vi "ACT_Loop.vi"() -> ()   [LabVIEW 2023, in "2024 AdPivotArm_ACT.lvlib"]
uses:
  2024 AdPivotArm_ACT.lvlib
  Cluster_CMD_ACT_Data.ctl
  Shared Code/TypeDefs/ENUM_Extend_CMD_Mode Select.ctl
  Shared Code/TypeDefs/Cluster_Extend_Config HW Values.ctl
  Shared Code/TypeDefs/Cluser_CAN Data.ctl
  Shared Code/TypeDefs/Cluster_Config FX Motor Output.ctl
  <vilib>/Rock Robotics/WPI/ThirdParty/Phoenix-LabVIEW/Motor Controller/Controls/CTRE_Phoenix_MotorControl_TalonFXInvertType.ctl
  <vilib>/Rock Robotics/WPI/ThirdParty/Phoenix-LabVIEW/Motor Controller/Controls/CTRE_Phoenix_MotorControl_NeutralMode.ctl
  Shared Code/TypeDefs/Cluster_FWD  REV Values.ctl
  Shared Code/TypeDefs/Cluster_FX SLOT PID Config.ctl
  Shared Code/TypeDefs/Cluster_PID Gains.ctl
  Shared Code/TypeDefs/Cluster_FX Motion Magic Parameters.ctl
  Shared Code/TypeDefs/Cluser_FX Config_Limit Travel.ctl
  Shared Code/TypeDefs/Cluser_Hard Limits.ctl
  <vilib>/Rock Robotics/WPI/ThirdParty/Phoenix-LabVIEW/Motor Controller/Controls/CTRE_Phoenix_MotorControl_LimitSwitchNormal.ctl
  Shared Code/TypeDefs/Cluser_Config_Soft Limits.ctl
  Shared Code/TypeDefs/Cluser_Enable-Value I32.ctl
  Shared Code/TypeDefs/Cluser_FX Config_Current Limits.ctl
  Shared Code/TypeDefs/Cluster_Cancoder_Config Data.ctl
  Shared Code/TypeDefs/Cluster_Extend HW Outputs.ctl
  Shared Code/TypeDefs/Cluster_FX CloseLoop Values.ctl
  Shared Code/TypeDefs/Cluster_FX Limit Switchs.ctl
  Shared Code/TypeDefs/Cluster_FX Current Values.ctl
  Shared Code/TypeDefs/Cluster_FX Sensor Values.ctl
  Shared Code/TypeDefs/Cluster_FX Integrated Sensor Values.ctl
  Shared Code/TypeDefs/Cluster_Extend_Config SW Values.ctl
  ENUM_ACT_State.ctl
  Shared Code/TypeDefs/Cluster_Extend_SW Output Data.ctl
  <vilib>/Rock Robotics/WPI/MotorControl/WPI_MotorControlDeviceRef.ctl
  <vilib>/Rock Robotics/WPI/MotorControl/WPI_MotorControlType.ctl
  <vilib>/Rock Robotics/SystemInterfaces/DIO/FPGA_DIOPWMChannel.ctl
  <vilib>/Rock Robotics/WPI/PWM/WPI_PWMDeadband.ctl
  <vilib>/Rock Robotics/SystemInterfaces/DIO/FPGA_DIOChannel.ctl
  <vilib>/Rock Robotics/WPI/ThirdParty/Phoenix-LabVIEW/Motor Controller/Controls/CTRE_Phoenix_MotorControl_ControlMode.ctl
  <vilib>/Rock Robotics/WPI/ThirdParty/Phoenix-LabVIEW/CANCoder/Controls/CTRE_Phoenix_CANcoder_DeviceRef.ctl
  ENUM_ACT_Action.ctl
  04ee53c9-9b63-4246-8662-e0753b0c7ce8.vi
  59f07e0f-2f3e-411b-a9d4-f777b7e34f70.vi
  d67cbdc1-c35e-4f58-b6c3-7121fa6e24ba.vi
  267fcfdb-c0dc-47c1-88bc-4cfe90507065.vi
  b5508d6c-c1cc-4273-80c5-2077d34e1483.vi
  5f725c2a-0ce1-4524-8967-e83b15fdce90.vi
  89b44e99-2ed6-4dfc-a998-459b3a1fdd77.vi
  6cc16fe4-e2d9-446e-a92a-5a1cdf729577.vi
  90b56285-4e1a-4408-995a-2e9e279006c2.vi
  <vilib>/Utility/error.llb/Trim Whitespace.vi
  5f725c2a-0ce1-4524-8967-e83b15fdce90.vi/958b2683-dd4b-41b7-8ed1-41c95f63cef0.vi
  5f725c2a-0ce1-4524-8967-e83b15fdce90.vi/95f5fa9b-6175-4b34-88ee-cece92c38279.vi
  89b44e99-2ed6-4dfc-a998-459b3a1fdd77.vi/958b2683-dd4b-41b7-8ed1-41c95f63cef0.vi
  89b44e99-2ed6-4dfc-a998-459b3a1fdd77.vi/95f5fa9b-6175-4b34-88ee-cece92c38279.vi
  6cc16fe4-e2d9-446e-a92a-5a1cdf729577.vi/958b2683-dd4b-41b7-8ed1-41c95f63cef0.vi
  6cc16fe4-e2d9-446e-a92a-5a1cdf729577.vi/95f5fa9b-6175-4b34-88ee-cece92c38279.vi
  90b56285-4e1a-4408-995a-2e9e279006c2.vi/958b2683-dd4b-41b7-8ed1-41c95f63cef0.vi
  90b56285-4e1a-4408-995a-2e9e279006c2.vi/95f5fa9b-6175-4b34-88ee-cece92c38279.vi
  <vilib>/Utility/error.llb/Trim Whitespace One-Sided.vi
  5f725c2a-0ce1-4524-8967-e83b15fdce90.vi/95f5fa9b-6175-4b34-88ee-cece92c38279.vi/1c6bd52c-bbca-4d4a-a290-93ea2703fded.vi
  5f725c2a-0ce1-4524-8967-e83b15fdce90.vi/95f5fa9b-6175-4b34-88ee-cece92c38279.vi/47c2b0d5-b5fa-444e-9535-611565d375db.vi
  89b44e99-2ed6-4dfc-a998-459b3a1fdd77.vi/95f5fa9b-6175-4b34-88ee-cece92c38279.vi/1c6bd52c-bbca-4d4a-a290-93ea2703fded.vi
  89b44e99-2ed6-4dfc-a998-459b3a1fdd77.vi/95f5fa9b-6175-4b34-88ee-cece92c38279.vi/47c2b0d5-b5fa-444e-9535-611565d375db.vi
  6cc16fe4-e2d9-446e-a92a-5a1cdf729577.vi/95f5fa9b-6175-4b34-88ee-cece92c38279.vi/1c6bd52c-bbca-4d4a-a290-93ea2703fded.vi
  6cc16fe4-e2d9-446e-a92a-5a1cdf729577.vi/95f5fa9b-6175-4b34-88ee-cece92c38279.vi/47c2b0d5-b5fa-444e-9535-611565d375db.vi
  90b56285-4e1a-4408-995a-2e9e279006c2.vi/95f5fa9b-6175-4b34-88ee-cece92c38279.vi/1c6bd52c-bbca-4d4a-a290-93ea2703fded.vi
  90b56285-4e1a-4408-995a-2e9e279006c2.vi/95f5fa9b-6175-4b34-88ee-cece92c38279.vi/47c2b0d5-b5fa-444e-9535-611565d375db.vi
  RoboRIO Utilities/Global_STOP.vi
  Global_CMD_ACT_Data In.vi
  <vilib>/Utility/Data Type/Get Type Information.vi
  Shared Code/Utility/RWA/RWA/File/RWA_PC FIle Read String.vi
  Shared Code/Utility/RWA/RWA/Read Write Anything/RWA_File String.vi
  Shared Code/Utility/RWA/RWA/File/RWA_PC File Write String.vi
  <vilib>/Rock Robotics/WPI/ThirdParty/Phoenix-LabVIEW/CANCoder/Set/CTRE_Phoenix_CANcoder_SetPosition.vi
  Global_ACT_Data Out.vi
  <vilib>/Comparison/Equal/Equal Functor/Equal Functor.lvclass
panel:
  in  "CMD Override":T1(tab)
  in  "Velocity":dbl(slide) scale=-0.3..0.3
  in  "Target Counts":i32
  in  "Positon GO":bool
  out "Current Time":timestamp
  out "SW Outputs":T2
  out "Sensor Read time":dbl format="%.3f"
  in  "Force Home":bool
  out "State":T3
  in  "SW Config":T4={"ExtendSW Ver"=0, "Home Speed (0-1)"=0.2, "Enable Current Limit On Homing"=FALSE, "At Position Delay(S)"=0.2}
  out "HW Outputs":T5
  in  "Read Saved Config":bool
  in  "Update Config":bool
  in  "HW Config":T11={"ExtendHW Ver"=0, "CAN"={"ID"=11, "Bus"=""}, "Output"={"Type"=enum."Counter-Clockwise", "Neutral"=enum."Override to Coast", "Max"={"FWD"=1.0, "REV"=-1.0}, "Min"={"FWD"=0.0, "REV"=0.0}, "OL Ramp Rate (S)"=0.0, "Dead Band"=0.0, "CL Ramp Rate (S)"=0.0}, "CL"={"Gains"={"P"=1.0, "I"=0.01, "D"=0.0, "F"=0.0}, "Error Allowed"=0.0, "I Zone"=0.0, "Peak Out 0-1"=10000.0, "Max I Accu"=-1000.0}, "MM"={"Cruise Velocity"=5000, "Acceleration"=5000}, "TravelLimits"={"Hard"={"FWD Switch Normal"=enum."Normally Open", "FWD On will Zero Encoder "=FALSE, "REV Switch Normal"=enum."Normally Open", "REV On will Zero Encoder "=FALSE}, "Soft"={"FWD"={"Enable"=FALSE, "Counts"=0}, "REV"={"Enable"=FALSE, "Counts"=0}}}, "StatorLimit"={"Enable"=FALSE, "Current Limit"=0.0, "Threshold Current"=0.0, "Threshold Time"=0.0}, "Cancoder"={"ID"=0, "CW(t) CCW(f)"=TRUE, "Zero Offset"=0.0}} {"TravelLimits"."Soft"."REV"."Counts" format="%#.0f"; "TravelLimits"."Soft"."FWD"."Counts" format="%#.0f"; "Output"."Min"."REV" format="%.2f"; "Output"."Min"."FWD" format="%.2f"; "Output"."Max"."REV" format="%.2f"; "Output"."Max"."FWD" format="%.2f"; "CL"."Gains"."F" format="%#.8f"; "CL"."Gains"."D" format="%#.8f"; "CL"."Gains"."I" format="%#.8f"; "CL"."Gains"."P" format="%#.8f"}
  out "CMD":T27
  out "Cycle Time (S)":dbl format="%.3g"
  # "Teleop or Auto"
  # "STOP"
  # "Tune Output\nto 1023 Max"
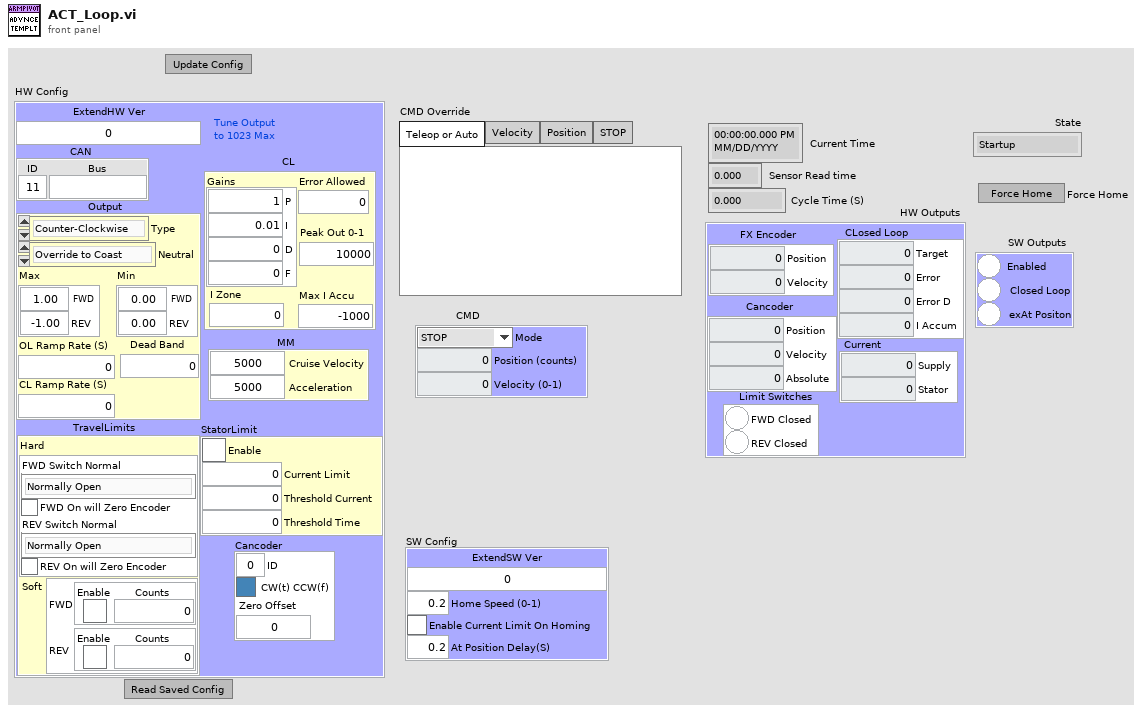
[diagram p1: front panel]
types:
  T1 = enum32{"Teleop or Auto", "Velocity", "Position", "STOP"}
  T2 = typedef "Cluster_Extend_SW Output Data.ctl" = cluster{"Enabled":bool, "Closed Loop":bool, "exAt Positon":bool}
  T3 = typedef "2024 AdPivotArm_ACT.lvlib/ENUM_ACT_State.ctl" = enum16{"Startup", "Configuring", "Stopping", "Moving Position", "Shutdown", "Homing", "Moving Velocity"}
  T4 = typedef "Cluster_Extend_Config SW Values.ctl" = cluster{"ExtendSW Ver":u64, "Home Speed (0-1)":dbl, "Enable Current Limit On Homing":bool, "At Position Delay(S)":dbl}
  T5 = typedef "Cluster_Extend HW Outputs.ctl" = cluster{"CLosed Loop":T6, "Limit Switches":T7, "Current":T8, "FX Encoder":T9, "Cancoder":T10}
  T6 = typedef "Cluster_FX CloseLoop Values.ctl" = cluster{"Target":dbl, "Error":i32, "Error D":dbl, "I Accum":dbl}
  T7 = typedef "Cluster_FX Limit Switchs.ctl" = cluster{"FWD Closed":bool, "REV Closed":bool}
  T8 = typedef "Cluster_FX Current Values.ctl" = cluster{"Supply":dbl, "Stator":dbl}
  T9 = typedef "Cluster_FX Sensor Values.ctl" = cluster{"Position":i32, "Velocity":i32}
  T10 = typedef "Cluster_FX Integrated Sensor Values.ctl" = cluster{"Position":dbl, "Velocity":dbl, "Absolute":dbl}
  T11 = typedef "Cluster_Extend_Config HW Values.ctl" = cluster{"ExtendHW Ver":u64, "CAN":T12, "Output":T13, "CL":T17, "MM":T19, "TravelLimits":T20, "StatorLimit":T25, "Cancoder":T26}
  T12 = typedef "Cluser_CAN Data.ctl" = cluster{"ID":u8, "Bus":string}
  T13 = typedef "Cluster_Config FX Motor Output.ctl" = cluster{"Type":T14, "Neutral":T15, "Max":T16, "Min":T16, "OL Ramp Rate (S)":dbl, "Dead Band":dbl, "CL Ramp Rate (S)":dbl}
  T14 = typedef "CTRE_Phoenix_MotorControl_TalonFXInvertType.ctl" = enum16{"Counter-Clockwise", "Clockwise"}
  T15 = typedef "CTRE_Phoenix_MotorControl_NeutralMode.ctl" = enum8{"EEPROMSetting", "Override to Coast", "Override to Brake"}
  T16 = typedef "Cluster_FWD  REV Values.ctl" = cluster{"FWD":dbl, "REV":dbl}
  T17 = typedef "Cluster_FX SLOT PID Config.ctl" = cluster{"Gains":T18, "Error Allowed":dbl, "I Zone":dbl, "Peak Out 0-1":dbl, "Max I Accu":dbl}
  T18 = typedef "Cluster_PID Gains.ctl" = cluster{"P":dbl, "I":dbl, "D":dbl, "F":dbl}
  T19 = typedef "Cluster_FX Motion Magic Parameters.ctl" = cluster{"Cruise Velocity":i32, "Acceleration":i32}
  T20 = typedef "Cluser_FX Config_Limit Travel.ctl" = cluster{"Hard":T21, "Soft":T23}
  T21 = typedef "Cluser_Hard Limits.ctl" = cluster{"FWD Switch Normal":T22, "FWD On will Zero Encoder ":bool, "REV Switch Normal":T22, "REV On will Zero Encoder ":bool}
  T22 = typedef "CTRE_Phoenix_MotorControl_LimitSwitchNormal.ctl" = enum16{"Normally Open", "Normally Closed", "Disabled"}
  T23 = typedef "Cluser_Config_Soft Limits.ctl" = cluster{"FWD":T24, "REV":T24}
  T24 = typedef "Cluser_Enable-Value I32.ctl" = cluster{"Enable":bool, "Counts":i32}
  T25 = typedef "Cluser_FX Config_Current Limits.ctl" = cluster{"Enable":bool, "Current Limit":dbl, "Threshold Current":dbl, "Threshold Time":dbl}
  T26 = typedef "Cluster_Cancoder_Config Data.ctl" = cluster{"ID":u8, "CW(t) CCW(f)":bool, "Zero Offset":dbl}
  T27 = typedef "2024 AdPivotArm_ACT.lvlib/Cluster_CMD_ACT_Data.ctl" = cluster{"Mode":T28, "Position (counts)":i32, "Velocity (0-1)":dbl}
  T28 = typedef "ENUM_Extend_CMD_Mode Select.ctl" = enum16{"STOP", "Position", "Velocity", "Force Home"}
  T29 = typedef "CTRE_Phoenix_CANcoder_DeviceRef.ctl" = cluster{"DeviceStatus":errorcluster, "Device Number":u8, "Handle":u64, "UsageFrame":u32, "Library Path":path}
  T30 = typedef "CTRE_Phoenix_MotorControl_ControlMode.ctl" = u16
  T31 = typedef "WPI_MotorControlDeviceRef.ctl" = cluster{"DeviceStatus":errorcluster, "Type":T32, "PWM":cluster{"PWM Channel":T33, "DeadBand":T34}, "CAN":cluster{"Device Number":u8, "SetOutput VI Ref":variant, "GetOutput VI Ref":variant, "Enable VI Ref":variant, "Disable VI Ref":variant, "Data":variant}, "Invert":bool, "DIO PWM":cluster{"PWM \"Enable\" Channel":T33, "DIOChannel":T35, "PWM Rate":dbl}}
  T32 = typedef "WPI_MotorControlType.ctl" = enum16{"PWM", "CAN", "DIO PWM"}
  T33 = typedef "FPGA_DIOPWMChannel.ctl" = enum8{"PWM 0", "PWM 1", "PWM 2", "PWM 3", "PWM 4", "PWM 5", "PWM 6", "PWM 7", "PWM 8", "PWM 9", "PWM MXP 0", "PWM MXP 1", "PWM MXP 2", "PWM MXP 3", "PWM MXP 4", "PWM MXP 5", "PWM MXP 6", "PWM MXP 7", "PWM MXP 8", "PWM MXP 9", "Invalid"}
  T34 = typedef "WPI_PWMDeadband.ctl" = cluster{"Name":string, "maxPositivePwm":i32, "minPositivePwm":i32, "centerPwm":i32, "maxNegativePwm":i32, "minNegativePwm":i32, "angularRange":u16}
  T35 = typedef "FPGA_DIOChannel.ctl" = enum8{"DIO 0", "DIO 1", "DIO 2", "DIO 3", "DIO 4", "DIO 5", "DIO 6", "DIO 7", "DIO 8", "DIO 9", "DIO MXP 0", "DIO MXP 1", "DIO MXP 2", "DIO MXP 3", "DIO MXP 4", "DIO MXP 5", "DIO MXP 6", "DIO MXP 7", "DIO MXP 8", "DIO MXP 9", "DIO MXP 10", "DIO MXP 11", "DIO MXP 12", "DIO MXP 13", "DIO MXP 14", "DIO MXP 15", "SPI Port CS1", "SPI Port CS2", "SPI Port CS3", "SPI Port MISO", "SPI Port MOSI", "Invalid"}
  T36 = cluster{"Falcon Ref":T31, "State":T3, "Previous State":T3, "Current Time":timestamp, "Previous Time":timestamp, "Start Time":timestamp, "Target Time (ms)":u32, "Cycle Time(S)":dbl, "ACT Input":T27, "ACT Output DBL":dbl, "Team Files Folder":path, "HW Config":T11, "Update Display":bool, "Max # Of Config Tries":i32, "CAN Timeout":u32, "FX Mode":T30, "FX Set Value":dbl, "HW Outputs":T5, "SW Config":T4, "SW Outputs":T2, "CANcoder Ref":T29, "Found Home":bool}
  T37 = typedef "2024 AdPivotArm_ACT.lvlib/ENUM_ACT_Action.ctl" = enum16{"No Action", "Reset Time", "Reset All", "Config HW File Read", "Config HW File Save", "Config SW File Read", "Config SW File Save", "Config From FP", "Config HW Extract", "Config HW Set", "Open HW Only", "Control FX Stop", "Control FX Home", "Control FX Motion Magic", "Control FX Speed", "Config Disable FX Soft Limit", "Config Enable FX Soft Limit", "Config HW Enable Current Limit", "Config HW Disable Current Limit", "Encoder Set to Zero", "Control FX Position", "Move to Reverse Limit "}
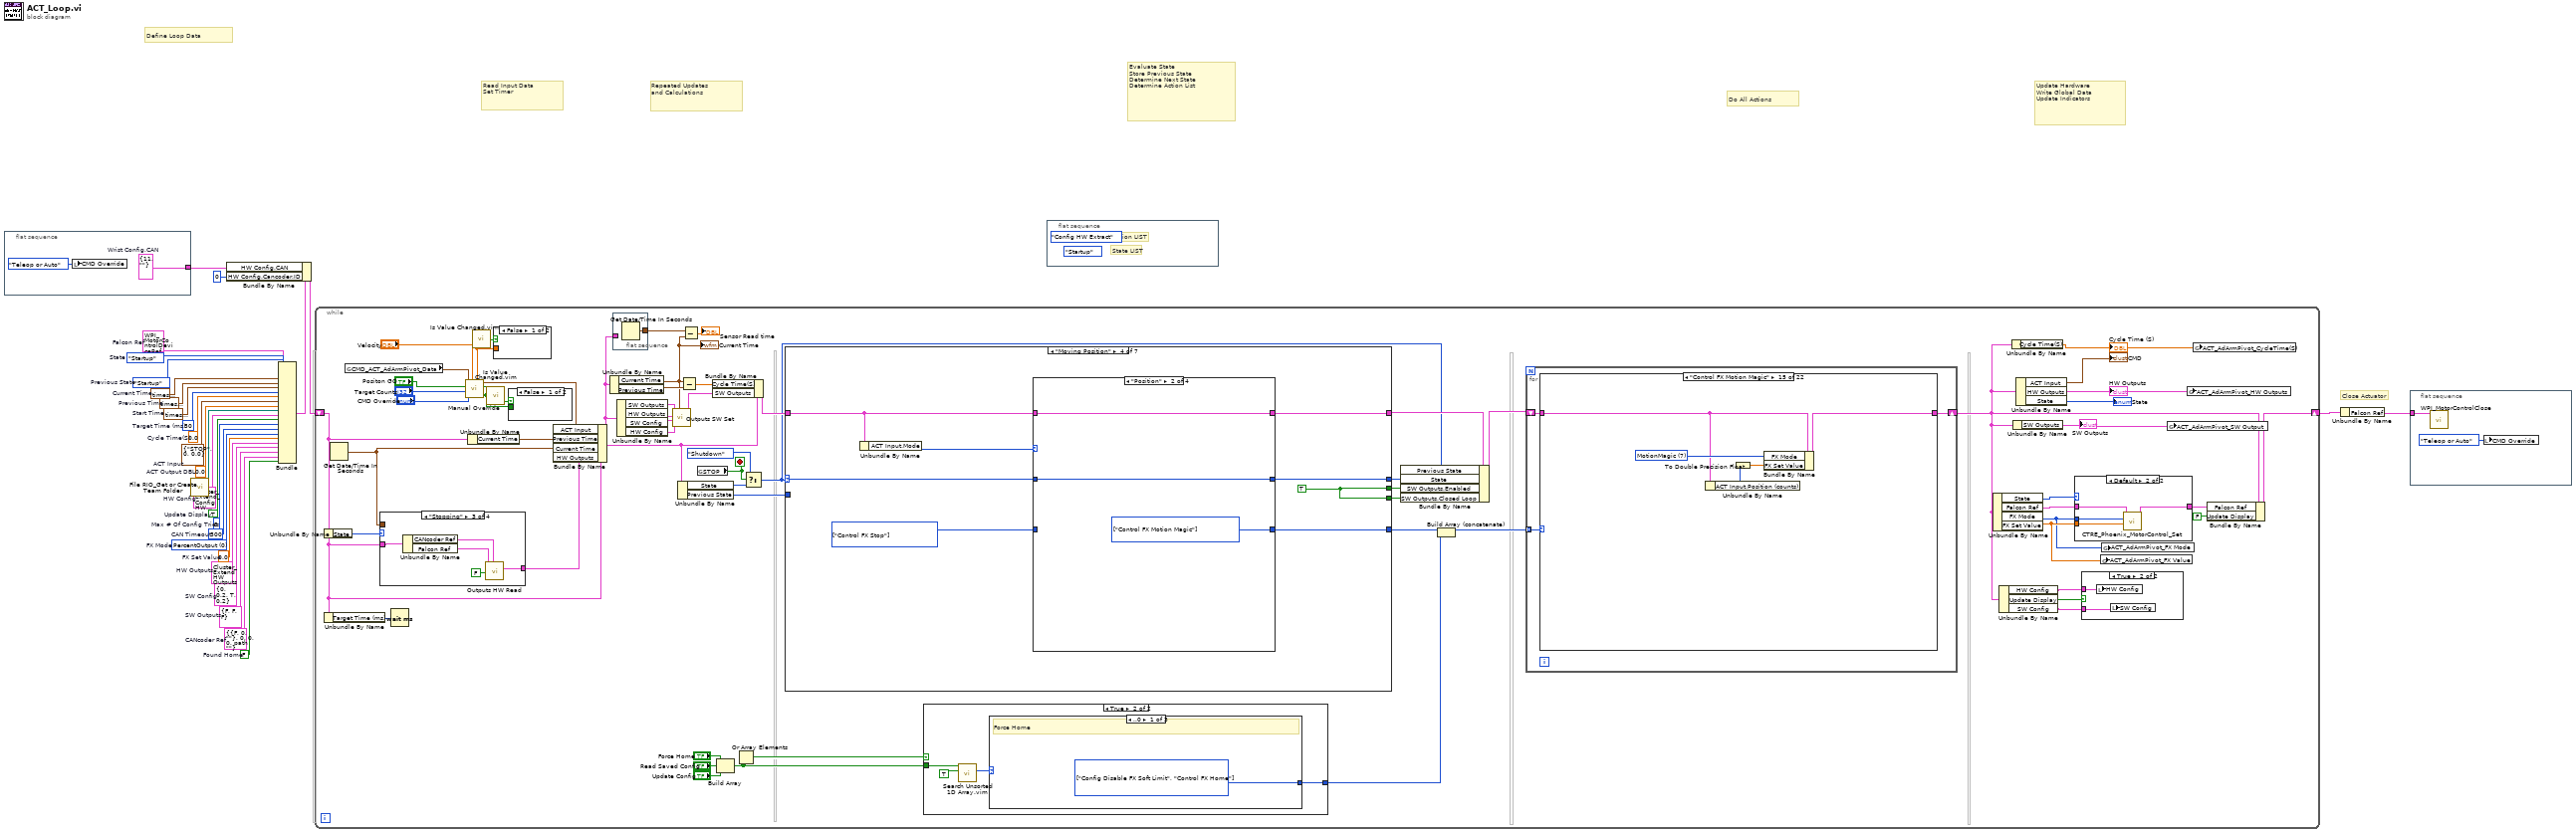
[diagram p0: block diagram]
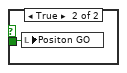
[diagram p2: hidden frame]
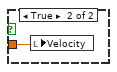
[diagram p3: hidden frame]
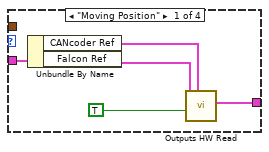
[diagram p4: hidden frame]
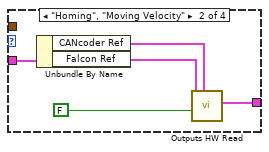
[diagram p5: hidden frame]
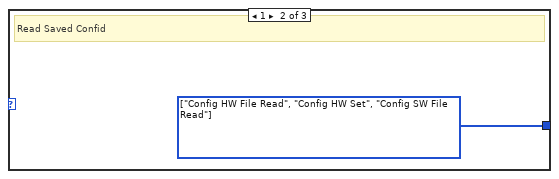
[diagram p8: hidden frame]
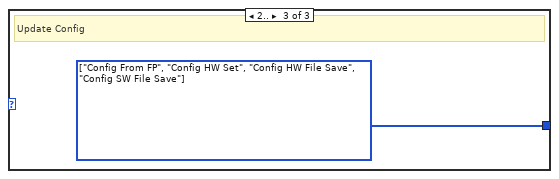
[diagram p9: hidden frame]
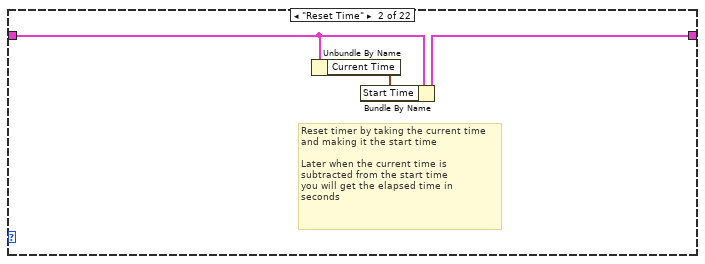
[diagram p13: hidden frame]
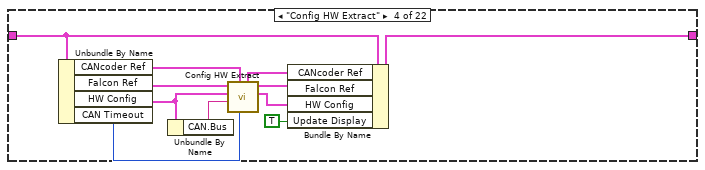
[diagram p15: hidden frame]
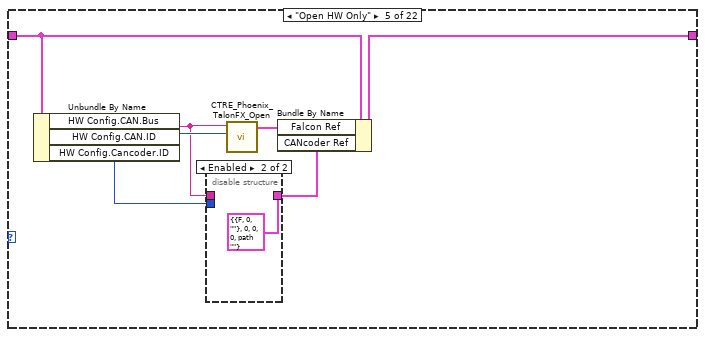
[diagram p16: hidden frame]
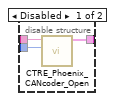
[diagram p17: hidden frame]
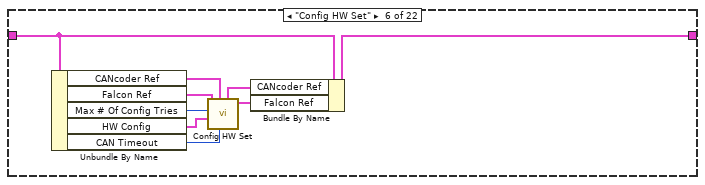
[diagram p18: hidden frame]
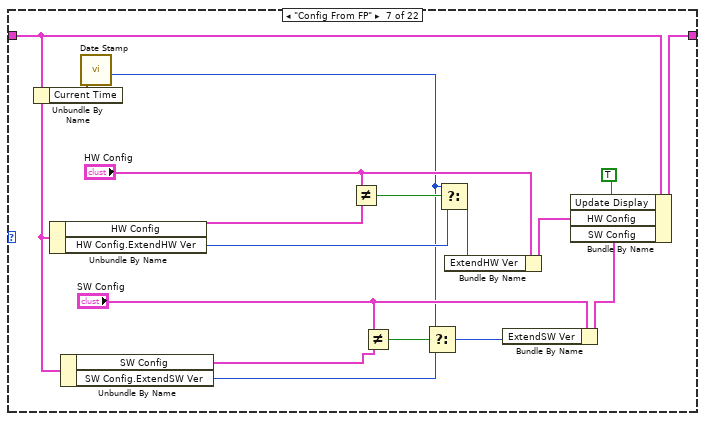
[diagram p19: hidden frame]
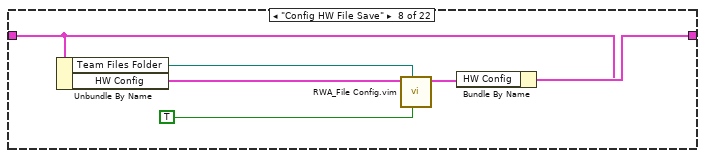
[diagram p20: hidden frame]
diagram:
  w1 = FALSE  # Found Home
  w3 = T29 {"DeviceStatus"={"status"=FALSE, "code"=0, "source"=""}, "Device Number"=0, "Handle"=0, "UsageFrame"=0, "Library Path"=path ""}  # CANcoder Ref
  w4 = T2 {"Enabled"=FALSE, "Closed Loop"=FALSE, "exAt Positon"=FALSE}  # SW Outputs
  w5 = T4 {"ExtendSW Ver"=0, "Home Speed (0-1)"=0.2, "Enable Current Limit On Homing"=TRUE, "At Position Delay(S)"=0.2}  # SW Config
  w6 = T5 {"CLosed Loop"={"Target"=0.0, "Error"=0, "Error D"=0.0, "I Accum"=0.0}, "Limit Switches"={"FWD Closed"=FALSE, "REV Closed"=FALSE}, "Current"={"Supply"=0.0, "Stator"=0.0}, "FX Encoder"={"Position"=0, "Velocity"=0}, "Cancoder"={"Position"=0.0, "Velocity"=0.0, "Absolute"=0.0}}  # HW Outputs
  w8 = 0.0  # FX Set Value
  w9 = T30 0 items=["PercentOutput"=0, "Position"=1, "Velocity"=2, "Current"=3, "Follower"=5, "MotionProfile"=6, "MotionMagic"=7, "MotionProfileArc"=10, "Disabled"=15]  # FX Mode
  w10 = u32 300  # CAN Timeout
  w11 = 3  # Max # Of Config Tries
  w12 = TRUE  # Update Display
  w14 = T11 {"ExtendHW Ver"=0, "CAN"={"ID"=0, "Bus"=""}, "Output"={"Type"=enum."Counter-Clockwise", "Neutral"=enum."EEPROMSetting", "Max"={"FWD"=0.0, "REV"=0.0}, "Min"={"FWD"=0.0, "REV"=0.0}, "OL Ramp Rate (S)"=0.0, "Dead Band"=0.0, "CL Ramp Rate (S)"=0.0}, "CL"={"Gains"={"P"=0.0, "I"=0.0, "D"=0.0, "F"=0.0}, "Error Allowed"=0.0, "I Zone"=0.0, "Peak Out 0-1"=0.0, "Max I Accu"=0.0}, "MM"={"Cruise Velocity"=0, "Acceleration"=0}, "TravelLimits"={"Hard"={"FWD Switch Normal"=enum."Normally Open", "FWD On will Zero Encoder "=FALSE, "REV Switch Normal"=enum."Normally Open", "REV On will Zero Encoder "=FALSE}, "Soft"={"FWD"={"Enable"=FALSE, "Counts"=0}, "REV"={"Enable"=FALSE, "Counts"=0}}}, "StatorLimit"={"Enable"=FALSE, "Current Limit"=0.0, "Threshold Current"=0.0, "Threshold Time"=0.0}, "Cancoder"={"ID"=0, "CW(t) CCW(f)"=FALSE, "Zero Offset"=0.0}}  # HW Config
  w16 = T31 {"DeviceStatus"={"status"=FALSE, "code"=0, "source"=""}, "Type"=enum."PWM", "PWM"={"PWM Channel"=enum."PWM 1", "DeadBand"={"Name"="", "maxPositivePwm"=0, "minPositivePwm"=0, "centerPwm"=0, "maxNegativePwm"=0, "minNegativePwm"=0, "angularRange"=0}}, "CAN"={"Device Number"=0, "SetOutput VI Ref"=variant(enum8{"Percent VBus", "Current", "Speed", "Position", "Voltage"} enum."Percent VBus"), "GetOutput VI Ref"=variant(refnum<k1> refnum), "Enable VI Ref"=variant(dbl 12.0), "Disable VI Ref"=variant(enum8{"Percent VBus", "Speed", "Position", "Slave", "Unchanged / Invalid", "Voltage Compensation", "Current", "Motion Profile"} enum."Percent VBus"), "Data"=variant}, "Invert"=FALSE, "DIO PWM"={"PWM \"Enable\" Channel"=enum."Invalid", "DIOChannel"=enum."Invalid", "PWM Rate"=0.0}}  # Falcon Ref
  w20 = 0.0  # Cycle Time(S)
  w21 = ENUM_ACT_State."Startup"  # Previous State
  w22 = timestamp(0 s since 1904-01-01)  # Previous Time
  w23 = u32 50  # Target Time (ms)
  w24 = 0.0  # ACT Output DBL
  w25 = T27 {"Mode"=enum."STOP", "Position (counts)"=0, "Velocity (0-1)"=0.0}  # ACT Input
  w26 = timestamp(0 s since 1904-01-01)  # Start Time
  w27 = timestamp(0 s since 1904-01-01)  # Current Time
  w28 = ENUM_ACT_State."Startup"  # State
  # "Close Actuator"
  # "Define Loop Data"
  # "Repeated Updates\nand Calculations"
  # "Read Input Data\nSet Timer"
  # "Evaluate State\nStore Previous State\nDetermine Next State\nDetermine Action List"
  # "Do All Actions"
  # "Update Hardware\nWrite Global Data\nUpdate Indicators"
  n1 = flat-sequence {
    tunnel: [w30] -> w13
    frame #0 {
      w30 = T12 {"ID"=11, "Bus"=""}  # Wrist Config.CAN
      n2 = local write "CMD Override"(T1."Teleop or Auto" ("CMD Override")) -> ()
    }
  }
  n3 = call "File RIO_Get or Create Team Folder.vi"() -> ("Team Files Folder"=w15:path)  [unwired: 10 in, 1 out]
  n4 = Bundle("Falcon Ref"=w16, "State"=w28, "Previous State"=w21, "Current Time"=w27, "Previous Time"=w22, "Start Time"=w26, "Target Time (ms)"=w23, "Cycle Time(S)"=w20, "ACT Input"=w25, "ACT Output DBL"=w24, "Team Files Folder"=w15, "HW Config"=w14, "Update Display"=w12, "Max # Of Config Tries"=w11, "CAN Timeout"=w10, "FX Mode"=w9, "FX Set Value"=w8, "HW Outputs"=w6, "SW Config"=w5, "SW Outputs"=w4, "CANcoder Ref"=w3, "Found Home"=w1) -> (w18:T36)  [unwired: 1 in]
  n5 = Bundle By Name(cluster=w18, "HW Config.CAN"=w13, "HW Config.Cancoder.ID"=u8 0) -> (w17:T36)
  n6 = while {
    shift-right: [w77] -> w19
    shift-left: w17 -> [w43]
    stop <- w89 stop-if-true
    n7 = Unbundle By Name(w43) -> ("State"=w69:T3)
    n8 = Unbundle By Name(w43) -> ("Target Time (ms)"=w86:u32)
    n9 = Get Date/Time In Seconds() -> (seconds since 1Jan1904=w55:timestamp)
    n10 = global read "Global_CMD_ACT_Data In.vi" "CMD_ACT_AdArmPivot_Data"() -> (w40:T27)
    n11 = case shown="\"Stopping\"" w69 {
      tunnel: w43 -> [w100 w105 w110 _]
      tunnel: w55 -> [_ _ _ _]
      tunnel: [w96 w101 w107 _] -> w44
      frame "Moving Position" {
        n12 = Unbundle By Name(w100) -> ("CANcoder Ref"=w97:T29, "Falcon Ref"=w99:T31)
        n13 = call "Outputs HW Read.vi"("CTRE_CANcoder_DeviceRef"=w97, "Read Closed Loop"=TRUE, "Ref"=w99) -> ("Sensor Values Out"=w96:T5)  [unwired: 5 in, 3 out]
      }
      frame "Homing", "Moving Velocity" {
        n14 = Unbundle By Name(w105) -> ("CANcoder Ref"=w102:T29, "Falcon Ref"=w104:T31)
        n15 = call "Outputs HW Read.vi"("CTRE_CANcoder_DeviceRef"=w102, "Read Closed Loop"=FALSE, "Ref"=w104) -> ("Sensor Values Out"=w101:T5)  [unwired: 5 in, 3 out]
      }
      frame "Stopping" {
        n16 = Unbundle By Name(w110) -> ("CANcoder Ref"=w108:T29, "Falcon Ref"=w109:T31)
        n17 = call "Outputs HW Read.vi"("CTRE_CANcoder_DeviceRef"=w108, "Read Closed Loop"=FALSE, "Ref"=w109) -> ("Sensor Values Out"=w107:T5)  [unwired: 5 in, 3 out]
      }
      frame "Startup", "Configuring", "Shutdown" {
      }
    }
    n18 = Wait (ms)(milliseconds to wait=w86) -> ()  [unwired: 1 out]
    n19 = call "Manual Override.vi"("Velocity"="Velocity", "Override"="CMD Override", "Counts"="Target Counts", "Position GO"="Positon GO", "Auto CMD"=w40) -> ("Position GO Out"=w35:bool, "OverRide Command Out"=w41:T27, "Velocity Out"=w37:dbl)  [unwired: 4 in]
    n20 = Unbundle By Name(w43) -> ("Current Time"=w85:timestamp)
    n21 = call "Is Value Changed.vim"("value"=w37) -> ("changed or first call?"=w36:bool)
    n22 = call "Is Value Changed.vim"("value"=w35) -> ("changed or first call?"=w34:bool)
    n23 = case shown="False" w36 {
      tunnel: w37 -> [_ w94]
      frame False {
      }
      frame True {
        n24 = local write "Velocity"(w94) -> ()
      }
    }
    n25 = case shown="False" w34 {
      tunnel: w35 -> [_ w93]
      frame False {
      }
      frame True {
        n26 = local write "Positon GO"(w93) -> ()
      }
    }
    n27 = Bundle By Name(cluster=w43, "ACT Input"=w41, "Previous Time"=w85, "Current Time"=w55, "HW Outputs"=w44) -> (w45:T36)
    n28 = Unbundle By Name(w45) -> ("Current Time"=w52:timestamp, "Previous Time"=w84:timestamp)
    "Current Time" <- w52
    n29 = flat-sequence {
      tunnel: [w95] -> w56
      tunnel: w45 -> [_]
      frame #0 {
        n30 = Get Date/Time In Seconds() -> (seconds since 1Jan1904=w95:timestamp)
      }
    }
    n31 = Unbundle By Name(w45) -> ("SW Outputs"=w51:T2, "HW Outputs"=w50:T5, "SW Config"=w49:T4, "HW Config"=w48:T11)
    n32 = call "Outputs SW Set.vi"("Current Time"=w52, "HW Config"=w48, "SW Config"=w49, "Sensor Values"=w50, "SW Output"=w51) -> ("SW Output Out"=w47:T2)  [unwired: 6 in]
    n33 = Unbundle By Name(w45) -> ("State"=w87:T3, "Previous State"=w46:T3)
    n34 = Subtract(x=w52, y=w84) -> (x-y=w82:dbl)
    n35 = Subtract(x=w56, y=w52) -> (x-y=→"Sensor Read time":dbl)
    n36 = global read "Global_STOP.vi" "STOP"() -> (w89:bool)
    n37 = Bundle By Name(cluster=w45, "Cycle Time(S)"=w82, "SW Outputs"=w47) -> (w83:T36)
    n38 = Build Array("Force Home", "Read Saved Config", "Update Config") -> (w60:bool[])
    n39 = Or Array Elements(Boolean array=w60) -> (logical OR=w61:bool)
    n40 = Select(t=ENUM_ACT_State."Shutdown" ("State"), s=w89, f=w87) -> (s? t:f=w67:T3)
    n41 = case shown="\"Moving Position\"" w67 {
      selector: w67 -> [_ _ _ w327 w348 _ w368]
      tunnel: w83 -> [w270 w274 w299 w329 w350 w366 w371]
      tunnel: [w270 w280 w304 w328 w349 w366 w370] -> w91
      tunnel: [ENUM_ACT_State."Configuring" ("State") w279 w303 w326 w347 ENUM_ACT_State."Shutdown" ("State") w372] -> w90
      tunnel: [w269 w278 w302 w324 w345 w364 w373] -> w81
      tunnel: w46 -> [_ _ _ _ _ _ w369]
      tunnel: [_ w271 TRUE w323 TRUE _ _] -> w32
      tunnel: [_ w271 TRUE w323 FALSE _ _] -> w31
      frame "Startup" {
        w269 = T37[] [enum."Reset Time"] items=["No Action", "Reset Time", "Reset All", "Config HW File Read", "Config HW File Save", "Config SW File Read", "Config SW File Save", "Config From FP", "Config HW Extract", "Config HW Set", "Open HW Only", "Control FX Stop", "Control FX Home", "Control FX Motion Magic", "Control FX Speed", "Config Disable FX Soft Limit", "Config Enable FX Soft Limit", "Config HW Enable Current Limit", "Config HW Disable Current Limit", "Encoder Set to Zero", "Control FX Position", "Move to Reverse Limit "] ("Actions")
      }
      frame "Configuring" {
        w271 = FALSE
        n42 = Unbundle By Name(w274) -> ("SW Config"=w276:T4)
        n43 = Unbundle By Name(w274) -> ("Team Files Folder"=w272:path, "HW Config"=w282:T11)
        n44 = call "Config_Build Name.vim"("Config First Name"=w276) -> ("Cfg file"=w277:string)  [unwired: 9 in, 1 out]
        n45 = call "Config_Build Name.vim"("Config First Name"=w282) -> ("Cfg file"=w284:string)  [unwired: 9 in, 1 out]
        n46 = Build Path(base path=w272, name or relative path=w277) -> (appended path=w275:path)
        n47 = call <vilib>:"Check if File or Folder Exists.vi"("path"=w275) -> ("file or folder exists?"=w273:bool)  [unwired: 8 in, 2 out]
        n48 = Build Path(base path=w272, name or relative path=w284) -> (appended path=w283:path)
        n49 = call <vilib>:"Check if File or Folder Exists.vi"("path"=w283) -> ("file or folder exists?"=w281:bool)  [unwired: 8 in, 2 out]
        n50 = case shown="True" w281 {
          tunnel: w274 -> [w287 w291]
          tunnel: [w287 w291] -> w280
          tunnel: [ENUM_ACT_State."Configuring" ("State") w290] -> w279
          tunnel: [w285 w289] -> w278
          tunnel: w273 -> [_ w288]
          frame False {
            w285 = T37[] [enum."Open HW Only", enum."Config HW Extract", enum."Config HW File Save"] items=["No Action", "Reset Time", "Reset All", "Config HW File Read", "Config HW File Save", "Config SW File Read", "Config SW File Save", "Config From FP", "Config HW Extract", "Config HW Set", "Open HW Only", "Control FX Stop", "Control FX Home", "Control FX Motion Magic", "Control FX Speed", "Config Disable FX Soft Limit", "Config Enable FX Soft Limit", "Config HW Enable Current Limit", "Config HW Disable Current Limit", "Encoder Set to Zero", "Control FX Position", "Move to Reverse Limit "] ("Actions")
            # "HW Config Not Found"
          }
          frame True {
            # "HW Config Found"
            n51 = case shown="True" w288 {
              tunnel: [ENUM_ACT_State."Configuring" ("State") ENUM_ACT_State."Homing" ("State")] -> w290
              tunnel: [w292 w294] -> w289
              frame False {
                w292 = T37[] [enum."Config SW File Save"] items=["No Action", "Reset Time", "Reset All", "Config HW File Read", "Config HW File Save", "Config SW File Read", "Config SW File Save", "Config From FP", "Config HW Extract", "Config HW Set", "Open HW Only", "Control FX Stop", "Control FX Home", "Control FX Motion Magic", "Control FX Speed", "Config Disable FX Soft Limit", "Config Enable FX Soft Limit", "Config HW Enable Current Limit", "Config HW Disable Current Limit", "Encoder Set to Zero", "Control FX Position", "Move to Reverse Limit "] ("Actions")
                # "SW Config NOT Found"
              }
              frame True {
                w294 = T37[] [enum."Config HW File Read", enum."Config HW Set", enum."Config SW File Read", enum."Reset All", enum."Control FX Stop"] items=["No Action", "Reset Time", "Reset All", "Config HW File Read", "Config HW File Save", "Config SW File Read", "Config SW File Save", "Config From FP", "Config HW Extract", "Config HW Set", "Open HW Only", "Control FX Stop", "Control FX Home", "Control FX Motion Magic", "Control FX Speed", "Config Disable FX Soft Limit", "Config Enable FX Soft Limit", "Config HW Enable Current Limit", "Config HW Disable Current Limit", "Encoder Set to Zero", "Control FX Position", "Move to Reverse Limit "] ("Actions")
                # "SW Config Found"
              }
            }
          }
        }
      }
      frame "Stopping" {
        n52 = Unbundle By Name(w299) -> ("ACT Input.Mode"=w305:T28)
        n53 = Unbundle By Name(w299) -> ("HW Outputs.Limit Switches.FWD Closed"=w298:bool, "HW Outputs.Limit Switches.REV Closed"=w297:bool)
        n54 = Or(x=w298, y=w297) -> (x .or. y?=w296:bool)
        n55 = case shown="True" w296 {
          tunnel: w305 -> [w310 _]
          tunnel: [w309 w322] -> w304
          tunnel: [w308 ENUM_ACT_State."Homing" ("State")] -> w303
          tunnel: [w307 w320] -> w302
          tunnel: w299 -> [w306 w322]
          frame False {
            n56 = case shown="\"Force Home\"" w310 {
              tunnel: w306 -> [w313 w315 w317 w319]
              tunnel: [w313 w315 w317 w319] -> w309
              tunnel: [ENUM_ACT_State."Stopping" ("State") ENUM_ACT_State."Homing" ("State") ENUM_ACT_State."Moving Position" ("State") ENUM_ACT_State."Moving Velocity" ("State")] -> w308
              tunnel: [w311 _ _ _] -> w307
              frame "STOP" {
                w311 = T37[] [enum."Control FX Stop"] items=["No Action", "Reset Time", "Reset All", "Config HW File Read", "Config HW File Save", "Config SW File Read", "Config SW File Save", "Config From FP", "Config HW Extract", "Config HW Set", "Open HW Only", "Control FX Stop", "Control FX Home", "Control FX Motion Magic", "Control FX Speed", "Config Disable FX Soft Limit", "Config Enable FX Soft Limit", "Config HW Enable Current Limit", "Config HW Disable Current Limit", "Encoder Set to Zero", "Control FX Position", "Move to Reverse Limit "] ("Actions")
              }
              frame "Force Home" {
              }
              frame "Position" {
              }
              frame "Velocity" {
              }
            }
          }
          frame True {
            w320 = T37[] [enum."Config Disable FX Soft Limit", enum."Control FX Home"] items=["No Action", "Reset Time", "Reset All", "Config HW File Read", "Config HW File Save", "Config SW File Read", "Config SW File Save", "Config From FP", "Config HW Extract", "Config HW Set", "Open HW Only", "Control FX Stop", "Control FX Home", "Control FX Motion Magic", "Control FX Speed", "Config Disable FX Soft Limit", "Config Enable FX Soft Limit", "Config HW Enable Current Limit", "Config HW Disable Current Limit", "Encoder Set to Zero", "Control FX Position", "Move to Reverse Limit "] ("Actions")
          }
        }
      }
      frame "Moving Position" {
        w323 = TRUE
        w325 = T37[] [enum."Control FX Stop"] items=["No Action", "Reset Time", "Reset All", "Config HW File Read", "Config HW File Save", "Config SW File Read", "Config SW File Save", "Config From FP", "Config HW Extract", "Config HW Set", "Open HW Only", "Control FX Stop", "Control FX Home", "Control FX Motion Magic", "Control FX Speed", "Config Disable FX Soft Limit", "Config Enable FX Soft Limit", "Config HW Enable Current Limit", "Config HW Disable Current Limit", "Encoder Set to Zero", "Control FX Position", "Move to Reverse Limit "] ("Actions")
        n57 = Unbundle By Name(w329) -> ("ACT Input.Mode"=w330:T28)
        n58 = case shown="\"Position\"" w330 {
          tunnel: w329 -> [w332 w336 w339 w342]
          tunnel: [w332 w336 w339 w342] -> w328
          tunnel: w327 -> [_ w335 _ _]
          tunnel: [ENUM_ACT_State."Stopping" ("State") w335 ENUM_ACT_State."Moving Velocity" ("State") ENUM_ACT_State."Homing" ("State")] -> w326
          tunnel: [w331 w334 w337 w340] -> w324
          tunnel: w325 -> [w331 _ w337 w340]
          frame "STOP" {
          }
          frame "Position" {
            w334 = T37[] [enum."Control FX Motion Magic"] items=["No Action", "Reset Time", "Reset All", "Config HW File Read", "Config HW File Save", "Config SW File Read", "Config SW File Save", "Config From FP", "Config HW Extract", "Config HW Set", "Open HW Only", "Control FX Stop", "Control FX Home", "Control FX Motion Magic", "Control FX Speed", "Config Disable FX Soft Limit", "Config Enable FX Soft Limit", "Config HW Enable Current Limit", "Config HW Disable Current Limit", "Encoder Set to Zero", "Control FX Position", "Move to Reverse Limit "] ("Actions")
          }
          frame "Velocity" {
          }
          frame "Force Home" {
          }
        }
      }
      frame "Moving Velocity" {
        w346 = T37[] [enum."Control FX Stop"] items=["No Action", "Reset Time", "Reset All", "Config HW File Read", "Config HW File Save", "Config SW File Read", "Config SW File Save", "Config From FP", "Config HW Extract", "Config HW Set", "Open HW Only", "Control FX Stop", "Control FX Home", "Control FX Motion Magic", "Control FX Speed", "Config Disable FX Soft Limit", "Config Enable FX Soft Limit", "Config HW Enable Current Limit", "Config HW Disable Current Limit", "Encoder Set to Zero", "Control FX Position", "Move to Reverse Limit "] ("Actions")
        n59 = Unbundle By Name(w350) -> ("ACT Input.Mode"=w351:T28)
        n60 = case shown="\"STOP\"" w351 {
          tunnel: w350 -> [w353 w356 w360 w363]
          tunnel: [w353 w356 w360 w363] -> w349
          tunnel: w348 -> [_ _ _ _]
          tunnel: [ENUM_ACT_State."Stopping" ("State") ENUM_ACT_State."Homing" ("State") ENUM_ACT_State."Moving Position" ("State") ENUM_ACT_State."Moving Velocity" ("State")] -> w347
          tunnel: [w352 w355 w358 w361] -> w345
          tunnel: w346 -> [w352 w355 w358 _]
          frame "STOP" {
          }
          frame "Force Home" {
          }
          frame "Position" {
          }
          frame "Velocity" {
            w361 = T37[] [enum."Control FX Speed"] items=["No Action", "Reset Time", "Reset All", "Config HW File Read", "Config HW File Save", "Config SW File Read", "Config SW File Save", "Config From FP", "Config HW Extract", "Config HW Set", "Open HW Only", "Control FX Stop", "Control FX Home", "Control FX Motion Magic", "Control FX Speed", "Config Disable FX Soft Limit", "Config Enable FX Soft Limit", "Config HW Enable Current Limit", "Config HW Disable Current Limit", "Encoder Set to Zero", "Control FX Position", "Move to Reverse Limit "] ("Actions")
          }
        }
      }
      frame "Shutdown" {
        w364 = T37[] [enum."Reset All"] items=["No Action", "Reset Time", "Reset All", "Config HW File Read", "Config HW File Save", "Config SW File Read", "Config SW File Save", "Config From FP", "Config HW Extract", "Config HW Set", "Open HW Only", "Control FX Stop", "Control FX Home", "Control FX Motion Magic", "Control FX Speed", "Config Disable FX Soft Limit", "Config Enable FX Soft Limit", "Config HW Enable Current Limit", "Config HW Disable Current Limit", "Encoder Set to Zero", "Control FX Position", "Move to Reverse Limit "] ("Actions")
      }
      frame "Homing" {
        n61 = Not Equal?(x=w368, y=w369) -> (x != y?=w367:bool)
        n62 = case shown="True" w367 {
          tunnel: [w382 w411] -> w373
          tunnel: [w381 w414] -> w372
          tunnel: w371 -> [w380 w410]
          tunnel: [w379 w413] -> w370
          tunnel: w368 -> [w374 w414]
          frame False {
            # "Not First Call"
            n63 = Unbundle By Name(w380) -> ("Found Home"=w375:bool, "HW Outputs.Limit Switches.FWD Closed"=w378:bool, "HW Outputs.Limit Switches.REV Closed"=w377:bool)
            n64 = Compound Arithmetic op=OR(w375, w378, w377) -> (w376:bool)
            n65 = case shown="True" w376 {
              tunnel: [w386 w401] -> w382
              tunnel: w374 -> [w387 _]
              tunnel: [w387 w394] -> w381
              tunnel: w380 -> [w384 w397]
              tunnel: [w385 w396] -> w379
              frame False {
                w386 = T37[] [enum."Config Disable FX Soft Limit", enum."Control FX Home"] items=["No Action", "Reset Time", "Reset All", "Config HW File Read", "Config HW File Save", "Config SW File Read", "Config SW File Save", "Config From FP", "Config HW Extract", "Config HW Set", "Open HW Only", "Control FX Stop", "Control FX Home", "Control FX Motion Magic", "Control FX Speed", "Config Disable FX Soft Limit", "Config Enable FX Soft Limit", "Config HW Enable Current Limit", "Config HW Disable Current Limit", "Encoder Set to Zero", "Control FX Position", "Move to Reverse Limit "] ("Actions")
                # "Not at home position"
                n66 = Unbundle By Name(w384) -> ("Current Time"=w383:timestamp)
                n67 = Bundle By Name(cluster=w384, "Start Time"=w383) -> (w385:T36)
              }
              frame True {
                w392 = 0.5  # Zero encoder timer
                # "At Home Positon or previously found home"
                n68 = Unbundle By Name(w397) -> ("Current Time"=w389:timestamp, "Start Time"=w390:timestamp, "HW Config.TravelLimits.Soft.FWD.Counts"=w388:i32, "HW Outputs.FX Encoder.Position"=w400:i32)
                n69 = Bundle By Name(cluster=w397, "Found Home"=TRUE) -> (w396:T36)
                n70 = Subtract(x=w389, y=w390) -> (x-y=w393:dbl)
                n71 = Greater?(x=w393, y=w392) -> (0:w391:bool)
                n72 = In Range and Coerce(upper limit=w388, x=w400, lower limit=-2000 ("upper limit")) -> (In Range?=w398:bool)  [unwired: 1 out]
                n73 = case shown="True" w398 {
                  tunnel: [w403 w406] -> w401
                  tunnel: [ENUM_ACT_State."Stopping" ("State") ENUM_ACT_State."Homing" ("State")] -> w394
                  tunnel: w391 -> [_ w404]
                  frame True {
                    w403 = T37[] [enum."Config Enable FX Soft Limit"] items=["No Action", "Reset Time", "Reset All", "Config HW File Read", "Config HW File Save", "Config SW File Read", "Config SW File Save", "Config From FP", "Config HW Extract", "Config HW Set", "Open HW Only", "Control FX Stop", "Control FX Home", "Control FX Motion Magic", "Control FX Speed", "Config Disable FX Soft Limit", "Config Enable FX Soft Limit", "Config HW Enable Current Limit", "Config HW Disable Current Limit", "Encoder Set to Zero", "Control FX Position", "Move to Reverse Limit "] ("Actions")
                    # "Extender is off of limit switch or zero"
                  }
                  frame False {
                    # "Extender is on limit switch"
                    n74 = case shown="False" w404 {
                      tunnel: [w407 w408] -> w406
                      frame False {
                        w407 = T37[] [enum."Encoder Set to Zero"] items=["No Action", "Reset Time", "Reset All", "Config HW File Read", "Config HW File Save", "Config SW File Read", "Config SW File Save", "Config From FP", "Config HW Extract", "Config HW Set", "Open HW Only", "Control FX Stop", "Control FX Home", "Control FX Motion Magic", "Control FX Speed", "Config Disable FX Soft Limit", "Config Enable FX Soft Limit", "Config HW Enable Current Limit", "Config HW Disable Current Limit", "Encoder Set to Zero", "Control FX Position", "Move to Reverse Limit "] ("Actions")
                        # "Reset timer not expired"
                      }
                      frame True {
                        w408 = T37[] [enum."Move to Reverse Limit "] items=["No Action", "Reset Time", "Reset All", "Config HW File Read", "Config HW File Save", "Config SW File Read", "Config SW File Save", "Config From FP", "Config HW Extract", "Config HW Set", "Open HW Only", "Control FX Stop", "Control FX Home", "Control FX Motion Magic", "Control FX Speed", "Config Disable FX Soft Limit", "Config Enable FX Soft Limit", "Config HW Enable Current Limit", "Config HW Disable Current Limit", "Encoder Set to Zero", "Control FX Position", "Move to Reverse Limit "] ("Actions")
                        # "Reset Timer expired"
                      }
                    }
                  }
                }
              }
            }
          }
          frame True {
            w411 = T37[] [enum."Config Disable FX Soft Limit", enum."Control FX Home"] items=["No Action", "Reset Time", "Reset All", "Config HW File Read", "Config HW File Save", "Config SW File Read", "Config SW File Save", "Config From FP", "Config HW Extract", "Config HW Set", "Open HW Only", "Control FX Stop", "Control FX Home", "Control FX Motion Magic", "Control FX Speed", "Config Disable FX Soft Limit", "Config Enable FX Soft Limit", "Config HW Enable Current Limit", "Config HW Disable Current Limit", "Encoder Set to Zero", "Control FX Position", "Move to Reverse Limit "] ("Actions")
            # "First call"
            n75 = Unbundle By Name(w410) -> ("Current Time"=w409:timestamp)
            n76 = Bundle By Name(cluster=w410, "Found Home"=FALSE, "Start Time"=w409) -> (w413:T36)
          }
        }
      }
    }
    n77 = case shown="True" w61 {
      tunnel: w60 -> [_ w114]
      tunnel: [_ w111] -> w59
      frame False {
      }
      frame True {
        n78 = call "Search Unsorted 1D Array.vim"("element"=TRUE, "unsorted 1D array"=w114) -> ("index of element"=w112:i32)  [unwired: 9 in]
        n79 = case shown="..0" w112 {
          tunnel: [w115 w116 w117] -> w111
          frame ..0 {
            w115 = T37[] [enum."Config Disable FX Soft Limit", enum."Control FX Home"] items=["No Action", "Reset Time", "Reset All", "Config HW File Read", "Config HW File Save", "Config SW File Read", "Config SW File Save", "Config From FP", "Config HW Extract", "Config HW Set", "Open HW Only", "Control FX Stop", "Control FX Home", "Control FX Motion Magic", "Control FX Speed", "Config Disable FX Soft Limit", "Config Enable FX Soft Limit", "Config HW Enable Current Limit", "Config HW Disable Current Limit", "Encoder Set to Zero", "Control FX Position", "Move to Reverse Limit "] ("Actions")
            # "Force Home"
          }
          frame 1 {
            w116 = T37[] [enum."Config HW File Read", enum."Config HW Set", enum."Config SW File Read"] items=["No Action", "Reset Time", "Reset All", "Config HW File Read", "Config HW File Save", "Config SW File Read", "Config SW File Save", "Config From FP", "Config HW Extract", "Config HW Set", "Open HW Only", "Control FX Stop", "Control FX Home", "Control FX Motion Magic", "Control FX Speed", "Config Disable FX Soft Limit", "Config Enable FX Soft Limit", "Config HW Enable Current Limit", "Config HW Disable Current Limit", "Encoder Set to Zero", "Control FX Position", "Move to Reverse Limit "] ("Actions")
            # "Read Saved Confid"
          }
          frame 2.. {
            w117 = T37[] [enum."Config From FP", enum."Config HW Set", enum."Config HW File Save", enum."Config SW File Save"] items=["No Action", "Reset Time", "Reset All", "Config HW File Read", "Config HW File Save", "Config SW File Read", "Config SW File Save", "Config From FP", "Config HW Extract", "Config HW Set", "Open HW Only", "Control FX Stop", "Control FX Home", "Control FX Motion Magic", "Control FX Speed", "Config Disable FX Soft Limit", "Config Enable FX Soft Limit", "Config HW Enable Current Limit", "Config HW Disable Current Limit", "Encoder Set to Zero", "Control FX Position", "Move to Reverse Limit "] ("Actions")
            # "Update Config"
          }
        }
      }
    }
    n80 = Bundle By Name(cluster=w91, "Previous State"=w67, "State"=w90, "SW Outputs.Enabled"=w32, "SW Outputs.Closed Loop"=w31) -> (w92:T36)
    n81 = Build Array (concatenate)(w81, w59) -> (w75:T37[])
    n82 = for {
      tunnel: w75 -> [w127] mode=indexing
      shift-right: [w126] -> w54
      shift-left: w92 -> [w125]
      n83 = case shown="\"Control FX Motion Magic\"" w127 {
        tunnel: w125 -> [w128 w131 w132 w139 w147 w161 w169 w185 w192 w198 w205 w209 w214 w218 w223 w230 w235 w240 w245 w253 w260 w264]
        tunnel: [w128 w130 w132 w140 w148 w162 w180 w186 w193 w199 w206 w210 w216 w220 w225 w232 w237 w241 w246 w254 w261 w265] -> w126
        frame "No Action" {
        }
        frame "Reset Time" {
          # "Reset timer by taking the current time\nand making it the start time\n\nLater when the current time is \nsubtracted from the start time\nyou will get the elapsed time in \nseconds"
          n84 = Unbundle By Name(w131) -> ("Current Time"=w129:timestamp)
          n85 = Bundle By Name(cluster=w131, "Start Time"=w129) -> (w130:T36)
        }
        frame "Reset All" {
        }
        frame "Config HW Extract" {
          n86 = Unbundle By Name(w139) -> ("CANcoder Ref"=w134:T29, "Falcon Ref"=w143:T31, "HW Config"=w142:T11, "CAN Timeout"=w135:u32)
          n87 = Unbundle By Name(w142) -> ("CAN.Bus"=w141:string)
          n88 = call "Config HW Extract.vi"("Send Cmd Timout(ms)"=w135, "CANcoderRef"=w134, "CAN.Bus"=w141, "HW Config"=w142, "Ref"=w143) -> ("HW Config Data Out"=w137:T11, "Ref Out"=w138:T31, "CANcoderRef Out"=w133:T29)  [unwired: 3 in, 1 out]
          n89 = Bundle By Name(cluster=w139, "CANcoder Ref"=w133, "Falcon Ref"=w138, "HW Config"=w137, "Update Display"=TRUE) -> (w140:T36)
        }
        frame "Open HW Only" {
          n90 = Unbundle By Name(w147) -> ("HW Config.CAN.Bus"=w145:string, "HW Config.CAN.ID"=w150:u8, "HW Config.Cancoder.ID"=w144:u8)
          n91 = disable-structure shown="Enabled" {
            disable-tunnel: [w153 T29 {"DeviceStatus"={"status"=FALSE, "code"=0, "source"=""}, "Device Number"=0, "Handle"=0, "UsageFrame"=0, "Library Path"=path ""} ("CTRE_CANcoder_DeviceRef")] -> w146
            disable-tunnel: w145 -> [w152 _]
            disable-tunnel: w144 -> [w151 _]
            frame Disabled {
              n92 = call <vilib>:"CTRE_Phoenix_CANcoder_Open.vi"("Device Number"=w151, "CAN Bus"=w152) -> ("CTRE_CANcoder_DeviceRef"=w153:T29)  [unwired: 8 in, 1 out]
            }
            frame Enabled {
            }
          }
          n93 = call <vilib>:"CTRE_Phoenix_TalonFX_Open.vi"("Device Number"=w150, "CAN Bus"=w145) -> ("PhoenixMotorControlDevRef"=w149:T31)  [unwired: 8 in, 1 out]
          n94 = Bundle By Name(cluster=w147, "Falcon Ref"=w149, "CANcoder Ref"=w146) -> (w148:T36)
        }
        frame "Config HW Set" {
          n95 = Unbundle By Name(w161) -> ("CANcoder Ref"=w157:T29, "Falcon Ref"=w163:T31, "Max # Of Config Tries"=w156:i32, "HW Config"=w159:T11, "CAN Timeout"=w158:u32)
          n96 = call "Config HW Set.vi"("Send Cmd Timout(ms)"=w158, "CANcoder Ref"=w157, "HW Config"=w159, "Max # Of Tries"=w156, "DevRef"=w163) -> ("DevRef Out Out"=w160:T31, "CANcoder Ref Out"=w155:T29)  [unwired: 4 in, 1 out]
          n97 = Bundle By Name(cluster=w161, "CANcoder Ref"=w155, "Falcon Ref"=w160) -> (w162:T36)
        }
        frame "Config From FP" {
          n98 = Unbundle By Name(w169) -> ("Current Time"=w178:timestamp)
          n99 = Unbundle By Name(w169) -> ("HW Config"=w173:T11, "HW Config.ExtendHW Ver"=w171:u64)
          n100 = Unbundle By Name(w169) -> ("SW Config"=w166:T4, "SW Config.ExtendSW Ver"=w176:u64)
          n101 = call "Date Stamp.vi"("Time"=w178) -> ("U64 Out"=w164:u64)  [unwired: 5 in, 1 out]
          n102 = Not Equal?(x="HW Config", y=w173) -> (x != y?=w172:bool)
          n103 = Not Equal?(x="SW Config", y=w166) -> (x != y?=w177:bool)
          n104 = Select(t=w164, s=w177, f=w176) -> (s? t:f=w175:u64)
          n105 = Select(t=w164, s=w172, f=w171) -> (s? t:f=w170:u64)
          n106 = Bundle By Name(cluster="HW Config", "ExtendHW Ver"=w170) -> (w168:T11)
          n107 = Bundle By Name(cluster="SW Config", "ExtendSW Ver"=w175) -> (w174:T4)
          n108 = Bundle By Name(cluster=w169, "Update Display"=TRUE, "HW Config"=w168, "SW Config"=w174) -> (w180:T36)
        }
        frame "Config HW File Save" {
          n109 = Unbundle By Name(w185) -> ("Team Files Folder"=w181:path, "HW Config"=w184:T11)
          n110 = call "RWA_File Config.vim"("Read(f) Save(t)"=TRUE ("Read(f) Write(t)"), "Target Folder Folder"=w181, "Any Config"=w184) -> ("Any Config Out"=w183:T11)  [unwired: 4 in, 4 out]
          n111 = Bundle By Name(cluster=w185, "HW Config"=w183) -> (w186:T36)
        }
        frame "Config SW File Read" {
          n112 = Unbundle By Name(w192) -> ("Team Files Folder"=w188:path, "SW Config"=w191:T4)
          n113 = call "RWA_File Config.vim"("Read(f) Save(t)"=FALSE ("Read(f) Write(t)"), "Target Folder Folder"=w188, "Any Config"=w191) -> ("Any Config Out"=w190:T4)  [unwired: 4 in, 4 out]
          n114 = Bundle By Name(cluster=w192, "SW Config"=w190, "Update Display"=TRUE) -> (w193:T36)
        }
        frame "Config SW File Save" {
          n115 = Unbundle By Name(w198) -> ("Team Files Folder"=w194:path, "SW Config"=w197:T4)
          n116 = call "RWA_File Config.vim"("Read(f) Save(t)"=TRUE ("Read(f) Write(t)"), "Target Folder Folder"=w194, "Any Config"=w197) -> ("Any Config Out"=w196:T4)  [unwired: 4 in, 4 out]
          n117 = Bundle By Name(cluster=w198, "SW Config"=w196) -> (w199:T36)
        }
        frame "Config HW File Read" {
          n118 = Unbundle By Name(w205) -> ("Team Files Folder"=w201:path, "HW Config"=w204:T11)
          n119 = call "RWA_File Config.vim"("Read(f) Save(t)"=FALSE ("Read(f) Write(t)"), "Target Folder Folder"=w201, "Any Config"=w204) -> ("Any Config Out"=w203:T11)  [unwired: 4 in, 4 out]
          n120 = Bundle By Name(cluster=w205, "HW Config"=w203, "Update Display"=TRUE) -> (w206:T36)
        }
        frame "Control FX Stop" {
          w208 = T30 0 items=["PercentOutput"=0, "Position"=1, "Velocity"=2, "Current"=3, "Follower"=5, "MotionProfile"=6, "MotionMagic"=7, "MotionProfileArc"=10, "Disabled"=15] ("FX Mode")
          n121 = Bundle By Name(cluster=w209, "FX Mode"=w208, "FX Set Value"=0.0) -> (w210:T36)
        }
        frame "Control FX Home" {
          w215 = T30 0 items=["PercentOutput"=0, "Position"=1, "Velocity"=2, "Current"=3, "Follower"=5, "MotionProfile"=6, "MotionMagic"=7, "MotionProfileArc"=10, "Disabled"=15] ("FX Mode")
          n122 = Unbundle By Name(w214) -> ("SW Config.Home Speed (0-1)"=w213:dbl)
          n123 = Absolute Value(x=w213) -> (abs(x)=w211:dbl)
          n124 = Bundle By Name(cluster=w214, "State"=ENUM_ACT_State."Homing", "FX Mode"=w215, "FX Set Value"=w211) -> (w216:T36)
        }
        frame "Control FX Speed" {
          w219 = T30 0 items=["PercentOutput"=0, "Position"=1, "Velocity"=2, "Current"=3, "Follower"=5, "MotionProfile"=6, "MotionMagic"=7, "MotionProfileArc"=10, "Disabled"=15] ("FX Mode")
          n125 = Unbundle By Name(w218) -> ("ACT Input.Velocity (0-1)"=w217:dbl)
          n126 = Bundle By Name(cluster=w218, "FX Mode"=w219, "FX Set Value"=w217) -> (w220:T36)
        }
        frame "Control FX Motion Magic" {
          w224 = T30 7 items=["PercentOutput"=0, "Position"=1, "Velocity"=2, "Current"=3, "Follower"=5, "MotionProfile"=6, "MotionMagic"=7, "MotionProfileArc"=10, "Disabled"=15] ("FX Mode")
          n127 = Unbundle By Name(w223) -> ("ACT Input.Position (counts)"=w222:i32)
          n128 = To Double Precision Float(number=w222) -> (double precision float=w221:dbl)
          n129 = Bundle By Name(cluster=w223, "FX Mode"=w224, "FX Set Value"=w221) -> (w225:T36)
        }
        frame "Move to Reverse Limit " {
          w231 = T30 1 items=["PercentOutput"=0, "Position"=1, "Velocity"=2, "Current"=3, "Follower"=5, "MotionProfile"=6, "MotionMagic"=7, "MotionProfileArc"=10, "Disabled"=15] ("FX Mode")
          n130 = Unbundle By Name(w230) -> ("HW Config.TravelLimits.Soft.FWD.Counts"=w229:i32)
          n131 = Subtract(x=w229, y=100) -> (x-y=w227:i32)
          n132 = To Double Precision Float(number=w227) -> (double precision float=w226:dbl)
          n133 = Bundle By Name(cluster=w230, "FX Mode"=w231, "FX Set Value"=w226) -> (w232:T36)
        }
        frame "Control FX Position" {
          w236 = T30 1 items=["PercentOutput"=0, "Position"=1, "Velocity"=2, "Current"=3, "Follower"=5, "MotionProfile"=6, "MotionMagic"=7, "MotionProfileArc"=10, "Disabled"=15] ("FX Mode")
          n134 = Unbundle By Name(w235) -> ("ACT Input.Position (counts)"=w234:i32)
          n135 = To Double Precision Float(number=w234) -> (double precision float=w233:dbl)
          n136 = Bundle By Name(cluster=w235, "FX Mode"=w236, "FX Set Value"=w233) -> (w237:T36)
        }
        frame "Config Disable FX Soft Limit" {
          n137 = Unbundle By Name(w240) -> ("Falcon Ref"=w242:T31)
          n138 = call <vilib>:"CTRE_Phoenix_MotorControl_OverrideSoftLimtsEnable.vi"("PhoenixMotorControlDevRef"=w242, "Override Soft Limit Enable?"=FALSE) -> ("PhoenixMotorControlDevRef"=w239:T31)  [unwired: 12 in, 1 out]
          n139 = Bundle By Name(cluster=w240, "Falcon Ref"=w239) -> (w241:T36)
        }
        frame "Config Enable FX Soft Limit" {
          n140 = Unbundle By Name(w245) -> ("Falcon Ref"=w247:T31)
          n141 = call <vilib>:"CTRE_Phoenix_MotorControl_OverrideSoftLimtsEnable.vi"("PhoenixMotorControlDevRef"=w247, "Override Soft Limit Enable?"=TRUE) -> ("PhoenixMotorControlDevRef"=w244:T31)  [unwired: 12 in, 1 out]
          n142 = Bundle By Name(cluster=w245, "Falcon Ref"=w244) -> (w246:T36)
        }
        frame "Config HW Disable Current Limit" {
          n143 = Unbundle By Name(w253) -> ("Falcon Ref"=w255:T31, "HW Config.StatorLimit"=w251:T25)
          n144 = Bundle By Name(cluster=w251, "Enable"=FALSE) -> (w249:T25)
          n145 = call <vilib>:"CTRE_Phoenix_MotorControl_ConfigStatorCurrentLimit.vi"("Stator Current Limit Configuration"=w249, "PhoenixMotorControlDevRef"=w255) -> ("PhoenixMotorControlDevRef"=w252:T31)  [unwired: 8 in, 1 out]
          n146 = Bundle By Name(cluster=w253, "Falcon Ref"=w252, "HW Config.StatorLimit"=w249, "Update Display"=TRUE) -> (w254:T36)
        }
        frame "Config HW Enable Current Limit" {
          n147 = Unbundle By Name(w260) -> ("Falcon Ref"=w262:T31, "HW Config.StatorLimit"=w258:T25)
          n148 = Bundle By Name(cluster=w258, "Enable"=TRUE) -> (w256:T25)
          n149 = call <vilib>:"CTRE_Phoenix_MotorControl_ConfigStatorCurrentLimit.vi"("Stator Current Limit Configuration"=w256, "PhoenixMotorControlDevRef"=w262) -> ("PhoenixMotorControlDevRef"=w259:T31)  [unwired: 8 in, 1 out]
          n150 = Bundle By Name(cluster=w260, "Falcon Ref"=w259, "HW Config.StatorLimit"=w256) -> (w261:T36)
        }
        frame "Encoder Set to Zero" {
          n151 = Unbundle By Name(w264) -> ("CANcoder Ref"=w266:T29)
          n152 = call-poly <vilib>:"CTRE_Phoenix_CANcoder_SetPositionPolymorphic.vi"("Position"=0.0, "CTRE_CANcoder_DeviceRef"=w266) -> ("CTRE_CANcoder_DeviceRef"=w263:T29)  [unwired: 8 in, 1 out]
          n153 = Bundle By Name(cluster=w264, "CANcoder Ref"=w263) -> (w265:T36)
        }
      }
    }
    n154 = Unbundle By Name(w54) -> ("State"=w70:T3, "Falcon Ref"=w79:T31, "FX Mode"=w71:T30, "FX Set Value"=w72:dbl)
    n155 = Unbundle By Name(w54) -> ("HW Config"=w73:T11, "Update Display"=w74:bool, "SW Config"=w66:T4)
    n156 = Unbundle By Name(w54) -> ("Cycle Time(S)"=w76:dbl)
    "Cycle Time (S)" <- w76
    n157 = Unbundle By Name(w54) -> ("SW Outputs"=w53:T2)
    "SW Outputs" <- w53
    n158 = Unbundle By Name(w54) -> ("ACT Input"=→"CMD":T27, "HW Outputs"=w68:T5, "State"=→"State":T3)
    "HW Outputs" <- w68
    n159 = case shown="Default" w70 {
      tunnel: w79 -> [w118 w122]
      tunnel: [w118 w121] -> w78
      tunnel: w72 -> [_ w120]
      tunnel: w71 -> [_ w119]
      frame "Startup", "Configuring" {
      }
      frame Default {
        n160 = call <vilib>:"CTRE_Phoenix_MotorControl_Set.vi"("Output"=w120, "Control Mode"=w119, "PhoenixMotorControlDevRef"=w122) -> ("PhoenixMotorControlDevRef"=w121:T31)  [unwired: 7 in, 1 out]
      }
    }
    n161 = case shown="True" w74 {
      tunnel: w73 -> [_ w124]
      tunnel: w66 -> [_ w123]
      frame False {
      }
      frame True {
        n162 = local write "HW Config"(w124) -> ()
        n163 = local write "SW Config"(w123) -> ()
      }
    }
    n164 = global write "Global_ACT_Data Out.vi" "ACT_AdArmPivot_FX Value"(w72) -> ()
    n165 = global write "Global_ACT_Data Out.vi" "ACT_AdArmPivot_FX Mode"(w71) -> ()
    n166 = global write "Global_ACT_Data Out.vi" "ACT_AdArmPivot_SW Output"(w53) -> ()
    n167 = global write "Global_ACT_Data Out.vi" "ACT_AdArmPivot_HW Outputs"(w68) -> ()
    n168 = global write "Global_ACT_Data Out.vi" "ACT_AdArmPivot_CycleTime(S)"(w76) -> ()
    n169 = Bundle By Name(cluster=w54, "Falcon Ref"=w78, "Update Display"=FALSE) -> (w77:T36)
  }
  n170 = flat-sequence {
    frame #0 {
      (unwired) ENUM_ACT_State."Startup" ("State")
      (unwired) ENUM_ACT_Action."Config HW Extract" ("Action")
      # "State LIST"
      # "Action LIST"
    }
  }
  n171 = Unbundle By Name(w19) -> ("Falcon Ref"=w7:T31)
  n172 = flat-sequence {
    tunnel: w7 -> [w416]
    frame #0 {
      n173 = call <vilib>:"WPI_MotorControlClose.vi"("MotorControlDevRef"=w416) -> ()  [unwired: 10 in, 1 out]
      n174 = local write "CMD Override"(T1."Teleop or Auto" ("CMD Override")) -> ()
    }
  }
